vi "Event_Structures.vi"() -> ()   [LabVIEW 2017]
panel:
  in  "RESET":bool
  in  "stop":bool
  out "String \nChanged":bool
  in  "String":string="Change me."
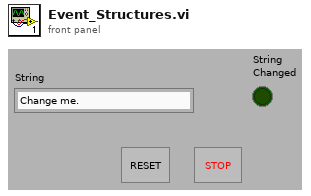
[diagram p1: front panel]
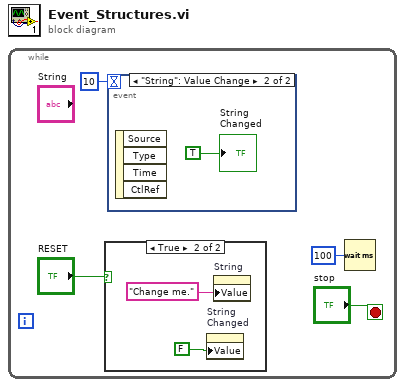
[diagram p0: block diagram]
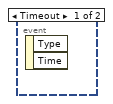
[diagram p2: hidden frame]
diagram:
  n1 = while {
    stop <- "stop" stop-if-true
    n2 = case shown="True" "RESET" {
      frame False {
      }
      frame True {
        n3 = property on="String \nChanged" class="Bool (strict)"("Value"=FALSE ("String Changed")) -> ()  [unwired: 2 in, 2 out]
        n4 = property on="String" class="Str"("Value"="Change me." ("String")) -> ()  [unwired: 2 in, 2 out]
      }
    }
    n5 = event shown="[1] \"String\": Value Change" {
      selector: _ -> [_ _]
      dyn-events: _ -> [_ _]
      timeout: 10 -> [_ _]
      event Timeout {
        n6 = event-data() -> ()  [unwired: 1 in, 2 out]
      }
      event "String": Value Change {
        n7 = event-data() -> ()  [unwired: 1 in, 4 out]
        "String \nChanged" <- TRUE ("String \nChanged")
      }
    }
    n8 = Wait (ms)(milliseconds to wait=u32 100) -> ()  [unwired: 1 out]
  }
